vi "Joystick Values To Joystick Data.vi"(0 "Xbox Name":string="Xbox", 1 "F310 Name":string="F310", 3 "Left X3D Joystick Name":string="My Joystick RefNum", 5 "Right X3D Joystick Name":string="My Joystick RefNum") -> ()   [LabVIEW 2020]
uses:
  Joystick Global 6740.vi
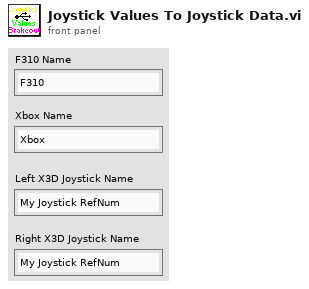
[diagram p1: front panel]
types:
  T1 = cluster{"A":bool, "B":bool, "X":bool, "Y":bool, "LB":bool, "RB":bool, "Back":bool, "Start":bool, "Left Joystick":bool, "Right Joystick":bool}
  T2 = cluster{"Left X":dbl, "Left Y":dbl, "Left Trigger":dbl, "Right Trigger":dbl, "Right X":dbl, "Right Y":dbl}
  T3 = cluster{"1":bool, "2":bool, "3":bool, "4":bool, "5":bool, "6":bool, "7":bool, "8":bool, "9":bool, "10":bool, "11":bool, "12":bool}
  T4 = cluster{"X Axis":dbl, "Y Axis":dbl, "Z Axis":dbl, "Slider":dbl}
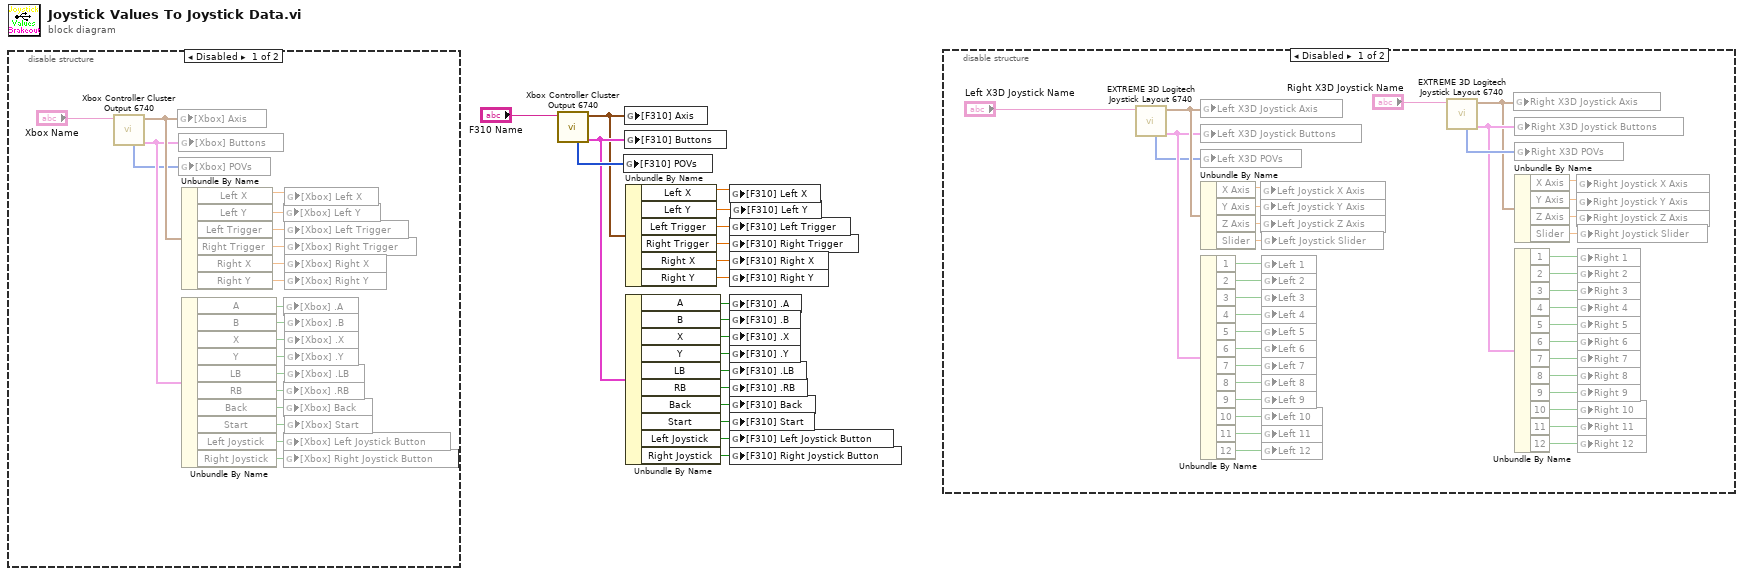
[diagram p0: block diagram]
diagram:
  n1 = disable-structure shown="Disabled" {
    frame Disabled {
      n2 = call "Xbox Controller Cluster Output 6740.vi"("Joystick Name"="Xbox Name") -> ("Buttons"=w23:T1, "Axis"=w24:T2, "POVs"=w21:i16[])  [unwired: 8 in]
      n3 = global write "Joystick Global 6740.vi" "[Xbox] Axis"(w24) -> ()
      n4 = global write "Joystick Global 6740.vi" "[Xbox] Buttons"(w23) -> ()
      n5 = global write "Joystick Global 6740.vi" "[Xbox] POVs"(w21) -> ()
      n6 = Unbundle By Name(w24) -> ("Left X"=w40:dbl, "Left Y"=w39:dbl, "Left Trigger"=w38:dbl, "Right Trigger"=w37:dbl, "Right X"=w36:dbl, "Right Y"=w35:dbl)
      n7 = Unbundle By Name(w23) -> ("A"=w34:bool, "B"=w33:bool, "X"=w32:bool, "Y"=w31:bool, "LB"=w30:bool, "RB"=w29:bool, "Back"=w28:bool, "Start"=w27:bool, "Left Joystick"=w26:bool, "Right Joystick"=w25:bool)
      n8 = global write "Joystick Global 6740.vi" "[Xbox] Left Y"(w39) -> ()
      n9 = global write "Joystick Global 6740.vi" "[Xbox] .A"(w34) -> ()
      n10 = global write "Joystick Global 6740.vi" "[Xbox] .RB"(w29) -> ()
      n11 = global write "Joystick Global 6740.vi" "[Xbox] Back"(w28) -> ()
      n12 = global write "Joystick Global 6740.vi" "[Xbox] Left Joystick Button"(w26) -> ()
      n13 = global write "Joystick Global 6740.vi" "[Xbox] Right Joystick Button"(w25) -> ()
      n14 = global write "Joystick Global 6740.vi" "[Xbox] Left X"(w40) -> ()
      n15 = global write "Joystick Global 6740.vi" "[Xbox] Left Trigger"(w38) -> ()
      n16 = global write "Joystick Global 6740.vi" "[Xbox] Right Trigger"(w37) -> ()
      n17 = global write "Joystick Global 6740.vi" "[Xbox] Right X"(w36) -> ()
      n18 = global write "Joystick Global 6740.vi" "[Xbox] Right Y"(w35) -> ()
      n19 = global write "Joystick Global 6740.vi" "[Xbox] .B"(w33) -> ()
      n20 = global write "Joystick Global 6740.vi" "[Xbox] .X"(w32) -> ()
      n21 = global write "Joystick Global 6740.vi" "[Xbox] .Y"(w31) -> ()
      n22 = global write "Joystick Global 6740.vi" "[Xbox] .LB"(w30) -> ()
      n23 = global write "Joystick Global 6740.vi" "[Xbox] Start"(w27) -> ()
    }
    frame Enabled {
    }
  }
  n24 = call "Xbox Controller Cluster Output 6740.vi"("Joystick Name"="F310 Name") -> ("Buttons"=w18:T1, "Axis"=w17:T2, "POVs"=w20:i16[])  [unwired: 8 in]
  n25 = global write "Joystick Global 6740.vi" "[F310] POVs"(w20) -> ()
  n26 = global write "Joystick Global 6740.vi" "[F310] Axis"(w17) -> ()
  n27 = global write "Joystick Global 6740.vi" "[F310] Buttons"(w18) -> ()
  n28 = Unbundle By Name(w17) -> ("Left X"=w1:dbl, "Left Y"=w2:dbl, "Left Trigger"=w3:dbl, "Right Trigger"=w4:dbl, "Right X"=w5:dbl, "Right Y"=w6:dbl)
  n29 = Unbundle By Name(w18) -> ("A"=w7:bool, "B"=w8:bool, "X"=w9:bool, "Y"=w10:bool, "LB"=w11:bool, "RB"=w12:bool, "Back"=w13:bool, "Start"=w14:bool, "Left Joystick"=w15:bool, "Right Joystick"=w16:bool)
  n30 = global write "Joystick Global 6740.vi" "[F310] Left X"(w1) -> ()
  n31 = global write "Joystick Global 6740.vi" "[F310] Left Trigger"(w3) -> ()
  n32 = global write "Joystick Global 6740.vi" "[F310] Right Trigger"(w4) -> ()
  n33 = global write "Joystick Global 6740.vi" "[F310] Right X"(w5) -> ()
  n34 = global write "Joystick Global 6740.vi" "[F310] Right Y"(w6) -> ()
  n35 = global write "Joystick Global 6740.vi" "[F310] .A"(w7) -> ()
  n36 = global write "Joystick Global 6740.vi" "[F310] .B"(w8) -> ()
  n37 = global write "Joystick Global 6740.vi" "[F310] .X"(w9) -> ()
  n38 = global write "Joystick Global 6740.vi" "[F310] .Y"(w10) -> ()
  n39 = global write "Joystick Global 6740.vi" "[F310] .LB"(w11) -> ()
  n40 = global write "Joystick Global 6740.vi" "[F310] .RB"(w12) -> ()
  n41 = global write "Joystick Global 6740.vi" "[F310] Back"(w13) -> ()
  n42 = global write "Joystick Global 6740.vi" "[F310] Start"(w14) -> ()
  n43 = global write "Joystick Global 6740.vi" "[F310] Left Joystick Button"(w15) -> ()
  n44 = global write "Joystick Global 6740.vi" "[F310] Right Joystick Button"(w16) -> ()
  n45 = global write "Joystick Global 6740.vi" "[F310] Left Y"(w2) -> ()
  n46 = disable-structure shown="Disabled" {
    frame Disabled {
      n47 = call "EXTREME 3D Logitech Joystick Layout 6740.vi"("Joystick Name"="Left X3D Joystick Name") -> ("Logitech Joystick Buttons"=w79:T3, "Logitech Joystick Axis"=w80:T4, "POVs"=w61:i16[])  [unwired: 8 in]
      n48 = global write "Joystick Global 6740.vi" "Left X3D Joystick Axis"(w80) -> ()
      n49 = global write "Joystick Global 6740.vi" "Left X3D Joystick Buttons"(w79) -> ()
      n50 = global write "Joystick Global 6740.vi" "Left X3D POVs"(w61) -> ()
      n51 = Unbundle By Name(w80) -> ("X Axis"=w78:dbl, "Y Axis"=w77:dbl, "Z Axis"=w76:dbl, "Slider"=w75:dbl)
      n52 = Unbundle By Name(w79) -> ("1"=w74:bool, "2"=w73:bool, "3"=w72:bool, "4"=w71:bool, "5"=w70:bool, "6"=w69:bool, "7"=w68:bool, "8"=w67:bool, "9"=w66:bool, "10"=w65:bool, "11"=w64:bool, "12"=w63:bool)
      n53 = global write "Joystick Global 6740.vi" "Left Joystick X Axis"(w78) -> ()
      n54 = global write "Joystick Global 6740.vi" "Left Joystick Y Axis"(w77) -> ()
      n55 = global write "Joystick Global 6740.vi" "Left Joystick Z Axis"(w76) -> ()
      n56 = global write "Joystick Global 6740.vi" "Left Joystick Slider"(w75) -> ()
      n57 = global write "Joystick Global 6740.vi" "Left 1"(w74) -> ()
      n58 = global write "Joystick Global 6740.vi" "Left 2"(w73) -> ()
      n59 = global write "Joystick Global 6740.vi" "Left 3"(w72) -> ()
      n60 = global write "Joystick Global 6740.vi" "Left 4"(w71) -> ()
      n61 = global write "Joystick Global 6740.vi" "Left 5"(w70) -> ()
      n62 = global write "Joystick Global 6740.vi" "Left 6"(w69) -> ()
      n63 = global write "Joystick Global 6740.vi" "Left 7"(w68) -> ()
      n64 = global write "Joystick Global 6740.vi" "Left 8"(w67) -> ()
      n65 = global write "Joystick Global 6740.vi" "Left 9"(w66) -> ()
      n66 = global write "Joystick Global 6740.vi" "Left 10"(w65) -> ()
      n67 = global write "Joystick Global 6740.vi" "Left 11"(w64) -> ()
      n68 = global write "Joystick Global 6740.vi" "Left 12"(w63) -> ()
      n69 = call "EXTREME 3D Logitech Joystick Layout 6740.vi"("Joystick Name"="Right X3D Joystick Name") -> ("Logitech Joystick Buttons"=w42:T3, "Logitech Joystick Axis"=w41:T4, "POVs"=w60:i16[])  [unwired: 8 in]
      n70 = global write "Joystick Global 6740.vi" "Right X3D Joystick Axis"(w41) -> ()
      n71 = global write "Joystick Global 6740.vi" "Right X3D Joystick Buttons"(w42) -> ()
      n72 = global write "Joystick Global 6740.vi" "Right X3D POVs"(w60) -> ()
      n73 = Unbundle By Name(w41) -> ("X Axis"=w43:dbl, "Y Axis"=w44:dbl, "Z Axis"=w45:dbl, "Slider"=w46:dbl)
      n74 = Unbundle By Name(w42) -> ("1"=w47:bool, "2"=w48:bool, "3"=w49:bool, "4"=w50:bool, "5"=w51:bool, "6"=w52:bool, "7"=w53:bool, "8"=w54:bool, "9"=w55:bool, "10"=w56:bool, "11"=w57:bool, "12"=w58:bool)
      n75 = global write "Joystick Global 6740.vi" "Right Joystick X Axis"(w43) -> ()
      n76 = global write "Joystick Global 6740.vi" "Right Joystick Y Axis"(w44) -> ()
      n77 = global write "Joystick Global 6740.vi" "Right Joystick Z Axis"(w45) -> ()
      n78 = global write "Joystick Global 6740.vi" "Right Joystick Slider"(w46) -> ()
      n79 = global write "Joystick Global 6740.vi" "Right 1"(w47) -> ()
      n80 = global write "Joystick Global 6740.vi" "Right 2"(w48) -> ()
      n81 = global write "Joystick Global 6740.vi" "Right 3"(w49) -> ()
      n82 = global write "Joystick Global 6740.vi" "Right 4"(w50) -> ()
      n83 = global write "Joystick Global 6740.vi" "Right 5"(w51) -> ()
      n84 = global write "Joystick Global 6740.vi" "Right 6"(w52) -> ()
      n85 = global write "Joystick Global 6740.vi" "Right 7"(w53) -> ()
      n86 = global write "Joystick Global 6740.vi" "Right 8"(w54) -> ()
      n87 = global write "Joystick Global 6740.vi" "Right 9"(w55) -> ()
      n88 = global write "Joystick Global 6740.vi" "Right 10"(w56) -> ()
      n89 = global write "Joystick Global 6740.vi" "Right 11"(w57) -> ()
      n90 = global write "Joystick Global 6740.vi" "Right 12"(w58) -> ()
    }
    frame Enabled {
    }
  }
